vi "Clear Read Buffer.vi"(8 "error in":errorcluster, 11 "connection ID":refnum<k5>) -> (0 "error out":errorcluster, 1 "bytes read":i32, 2 "data out":string, 3 "connection ID out":refnum<k5>, 4 "hex bytes":string)   [LabVIEW 2024]
uses:
  <vilib>/Utility/error.llb/Error Cluster From Error Code.vi
  <vilib>/ErrorRing/Error Ring.xnode
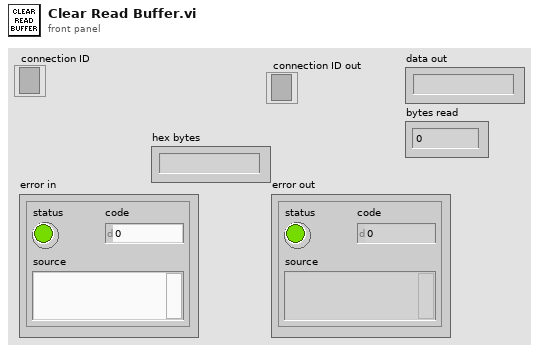
[diagram p1: front panel]
types:
  T1 = enum16{"Standard", "Buffered", "CRLF", "Immediate"}
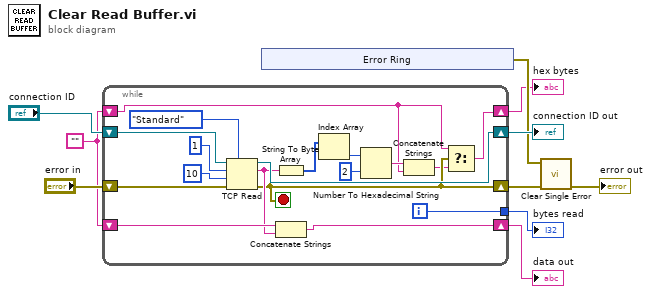
[diagram p0: block diagram]
diagram:
  w2 = ""
  n1 = while {
    shift-right: [w15] -> w7
    shift-left: "error in" -> [w24]
    shift-right: [w27] -> w10
    shift-left: "connection ID" -> [w23]
    shift-right: [w21] -> w4
    shift-left: w2 -> [w22]
    tunnel: [w20] -> w3
    shift-right: [w12] -> w1
    shift-left: w2 -> [w14]
    i -> [w20]
    stop <- w15 stop-if-true
    n2 = TCP Read(connection ID=w23, bytes to read=1, error in (no error)=w24, 7:T1."Standard" ("mode (standard)"), 9:10 ("timeout ms (25000)")) -> (connection ID out=w27:refnum<k5>, data out=w19:string, error out=w15:errorcluster)
    n3 = String To Byte Array(string=w19) -> (unsigned byte array=w18:u8[])
    n4 = Concatenate Strings(w22, w19) -> (w21:string)
    n5 = Index Array(array=w18) -> (element=w17:u8)  [unwired: 1 in]
    n6 = Number To Hexadecimal String(1:i16 2 ("width (-)"), 2:w17) -> (0:w16:string)
    n7 = Concatenate Strings(w16, w14) -> (w13:string)
    n8 = Select(t=w14, s=w15, f=w13) -> (s? t:f=w12:string)
  }
  "connection ID out" <- w10
  "data out" <- w4
  "bytes read" <- w3
  "hex bytes" <- w1
  n9 = xnode "Error Ring"() -> ("error out"=w5:errorcluster)
  n10 = call "Clear Single Error.vi"("Error In"=w7, "Error to clear"=w5) -> ("Error Out"=→"error out":errorcluster)  [unwired: 8 in, 1 out]
